vi "Read Velocity.vi"(11 "Movable in":refnum<class "Movable.lvclass">) -> (2 "Velocity":T1)   [LabVIEW 2024, in "Movable.lvclass"]
doc: "MIT Licence\nCopyright (c) 2024 David Grollier"
uses:
  Movable.lvclass
  Type Def/Velocity.ctl
  Movable.lvclass/Movable.ctl
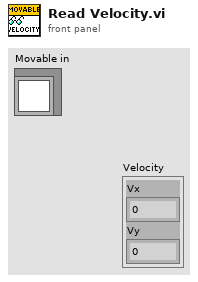
[diagram p1: front panel]
types:
  T1 = typedef "Velocity.ctl" = cluster{"Vx":dbl, "Vy":dbl}
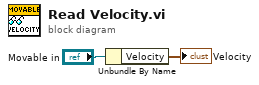
[diagram p0: block diagram]
diagram:
  n1 = Unbundle By Name("Movable in") -> ("Velocity"=→"Velocity":T1)
